vi "Import Transactions.vi"(8 "error in (no error)":errorcluster, 10 "Importing Transactions":refnum<class "Statement.lvclass">, 11 "Budgetizer in":refnum<class "Budgetizer.lvclass">) -> (0 "error out":errorcluster, 3 "Budgetizer out":refnum<class "Budgetizer.lvclass">)   [LabVIEW 2018, in "Budgetizer.lvclass"]
uses:
  Budgetizer.lvclass
  Statement/Statement.lvclass
  Budgetizer.lvclass/Budgetizer.ctl
  database/Database.lvclass
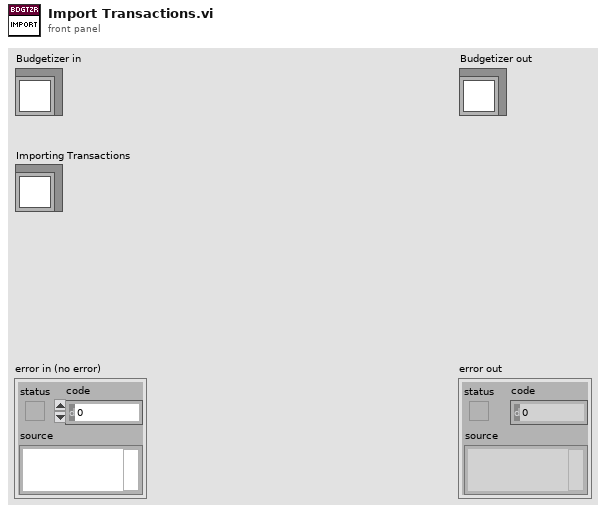
[diagram p1: front panel]
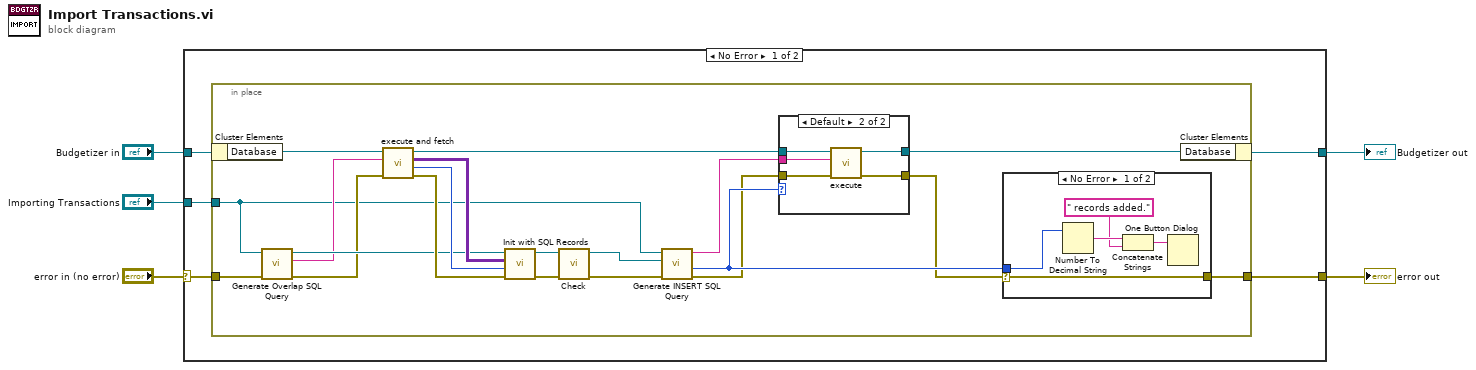
[diagram p0: block diagram]
diagram:
  n1 = case shown="No Error" "error in (no error)" {
    selector: "error in (no error)" -> [w10 w45]
    tunnel: [w9 w45] -> w4
    tunnel: [w6 w44] -> w2
    tunnel: "Budgetizer in" -> [w7 w44]
    tunnel: "Importing Transactions" -> [w8 _]
    frame No Error {
      n2 = in-place {
        in-place-border: w10 -> [w13]
        in-place-border: [w14] -> w9
        in-place-border: w8 -> [w12]
        n3 = in-place-cluster #1(w7) -> ("Database"=w22:refnum<class "Database.lvclass">)
        n4 = call-dynamic "Generate Overlap SQL Query.vi"("error in (no error)"=w13, "Importing Transactions"=w12) -> ("error out"=w23:errorcluster, "Overlap Query"=w24:string, "Overlapping Records"=w25:refnum<class "Statement.lvclass">)  [unwired: 7 in]
        n5 = call "execute and fetch.vi"("error in (no error)"=w23, "SQL query"=w24, "Database in"=w22) -> ("error out"=w26:errorcluster, "Num records"=w28:i32, "recordset data"=w27:variant[][], "Database out"=w16:refnum<class "Database.lvclass">)  [unwired: 5 in]
        n6 = call-dynamic "Init with SQL Records.vi"("error in (no error)"=w26, "Num records"=w28, "SQL Dataset"=w27, "Statement in"=w25) -> ("error out"=w30:errorcluster, "Statement out"=w29:refnum<class "Statement.lvclass">)  [unwired: 6 in]
        n7 = call-dynamic "Check.vi"("error in (no error)"=w30, "Statement in"=w29) -> ("error out"=w17:errorcluster, "Statement out"=w11:refnum<class "Statement.lvclass">)  [unwired: 8 in]
        n8 = call-dynamic "Generate INSERT SQL Query.vi"("error in (no error)"=w17, "Overlappping Records"=w11, "Importing Transactions"=w12) -> ("error out"=w18:errorcluster, "Num Recs to Insert"=w20:i32, "INSERT Query"=w21:string)  [unwired: 6 in]
        n9 = case shown="Default" w20 {
          tunnel: w16 -> [w32 w37]
          tunnel: [w32 w36] -> w15
          tunnel: w18 -> [w31 w35]
          tunnel: [w31 w33] -> w19
          tunnel: w21 -> [_ w34]
          frame 0 {
          }
          frame Default {
            n10 = call "execute.vi"("error in (no error)"=w35, "SQL query"=w34, "Database in"=w37) -> ("error out"=w33:errorcluster, "Database out"=w36:refnum<class "Database.lvclass">)  [unwired: 7 in]
          }
        }
        n11 = case shown="No Error" w19 {
          selector: w19 -> [w39 w43]
          tunnel: [w39 w43] -> w14
          tunnel: w20 -> [w38 _]
          frame No Error {
            n12 = Number To Decimal String(number=w38) -> (decimal integer string=w41:string)  [unwired: 1 in]
            n13 = Concatenate Strings(w41, " records added.") -> (w42:string)
            n14 = One Button Dialog(message=w42) -> ()  [unwired: 1 in, 1 out]
          }
          frame Error {
          }
        }
        n15 = in-place-cluster #1("Database"=w15) -> (w6:refnum<class "Budgetizer.lvclass">)
      }
    }
    frame Error {
    }
  }
  "error out" <- w4
  "Budgetizer out" <- w2
